vi "ACT_LabVIEW3_Task2_Team072.vi"() -> ()   [LabVIEW 2016]
uses:
  <vilib>/express/express arith-compare/Formula/XNode/ExpressFormulaBlockNode.xnode
panel:
  out "Output":dbl
  in  "End":dbl
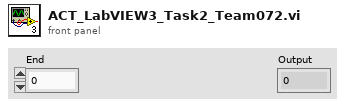
[diagram p1: front panel]
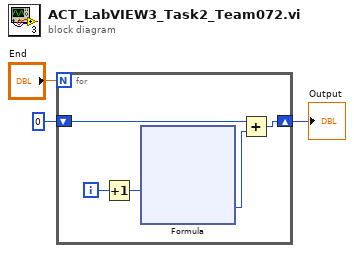
[diagram p0: block diagram]
diagram:
  n1 = for {
    N: "End" -> [_]
    shift-right: [w6] -> w1
    shift-left: 0 -> [w7]
    i -> [w5]
    n2 = Increment(x=w5) -> (x+1=w4:i32)
    n3 = xnode "Formula"("i"=w4) -> ("Result"=w8:i32)  [unwired: 1 in, 1 out]
    n4 = Add(x=w7, y=w8) -> (x+y=w6:i32)
  }
  "Output" <- w1
